vi "Demo_DatabaseTest_NIbase.vi"() -> ()   [LabVIEW 2016]
uses:
  <vilib>/addons/database/Connection.llb/DB Tools Open Connec (String).vi
  <vilib>/addons/database/Connection.llb/DB Tools Open Connec (Path).vi
  <vilib>/addons/database/Connection.llb/Conn Execute.vi
  <vilib>/addons/database/NI_Database_API.lvlib
panel:
  out "error out":errorcluster
  in  "msgid":dbl
  in  "content":string
  in  "dataLabel":string
  in  "TestId":string
  in  "错误输入 16":errorcluster caption="错误输入"
  in  "Connection Method":u16(ring) items=["ODBC System DSN", "UDL File", "Prompt"]
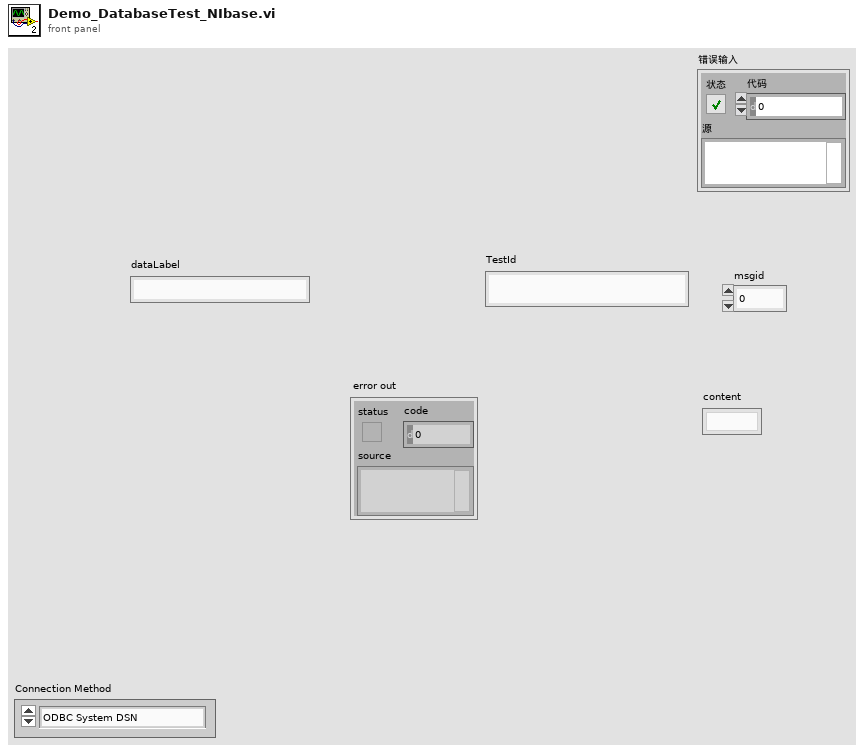
[diagram p1: front panel]
types:
  T1 = typedef "NI_Database_API.lvlib/Conn ObjectReference.ctl" = refnum<k1>
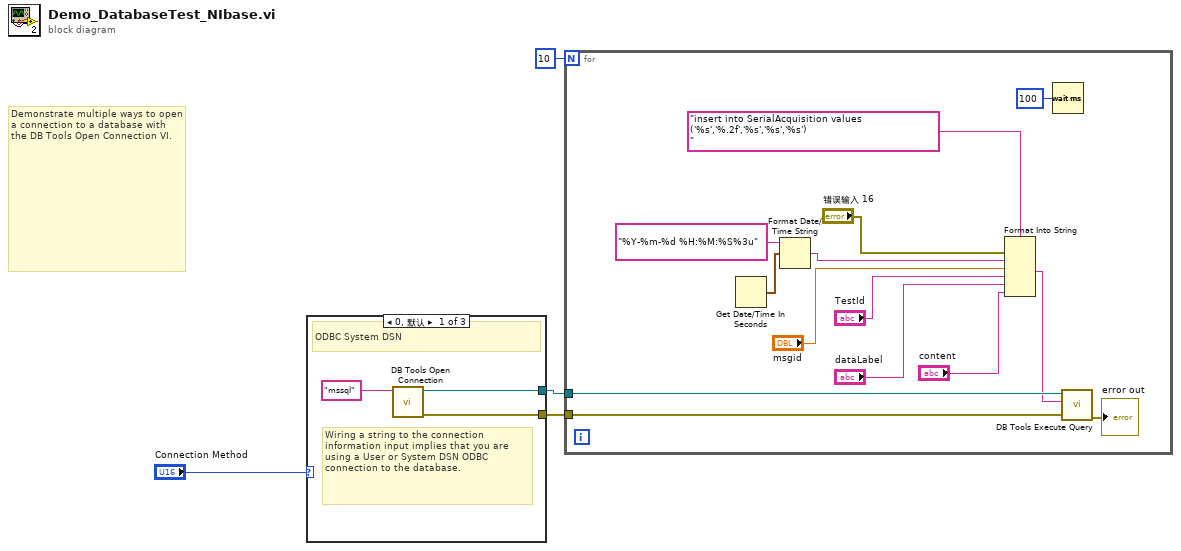
[diagram p0: block diagram]
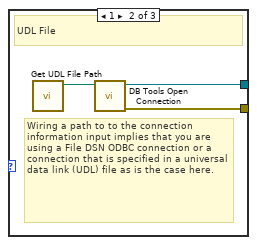
[diagram p2: hidden frame]
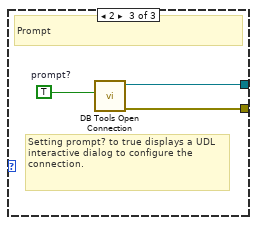
[diagram p3: hidden frame]
diagram:
  # "Demonstrate multiple ways to open a connection to a database with the DB Tools Open Connection VI."
  n1 = case shown="0, 默认" "Connection Method" {
    tunnel: [w6 w9 w13] -> w3
    tunnel: [w5 w10 w12] -> w2
    frame 0, Default {
      # "Wiring a string to the connection information input implies that you are using a User or System DSN ODBC connection to the database."
      # "ODBC System DSN"
      n2 = call-poly <vilib>:"DB Tools Open Connection.vi"("connection information"="mssql") -> ("error out"=w5:errorcluster, "connection reference"=w6:T1)  [unwired: 7 in]
    }
    frame 1 {
      # "Wiring a path to to the connection information input implies that you are using a File DSN ODBC connection or a connection that is specified in a universal data link (UDL) file as is the case here."
      # "UDL File"
      n3 = call "Get UDL File Path.vi"() -> ("UDL file path"=w8:path)  [unwired: 11 in]
      n4 = call-poly <vilib>:"DB Tools Open Connection.vi"("connection information"=w8) -> ("error out"=w10:errorcluster, "connection reference"=w9:T1)  [unwired: 7 in]
    }
    frame 2 {
      w11 = TRUE  # prompt?
      # "Setting prompt? to true displays a UDL interactive dialog to configure the connection."
      # "Prompt"
      n5 = call-poly <vilib>:"DB Tools Open Connection.vi"("prompt? (F)"=w11) -> ("error out"=w12:errorcluster, "connection reference"=w13:T1)  [unwired: 7 in]
    }
  }
  n6 = for {
    N: 10 -> [_]
    tunnel: w3 -> [w27]
    tunnel: w2 -> [w17]
    n7 = Get Date/Time In Seconds() -> (seconds since 1Jan1904=w24:timestamp)
    n8 = Format Date/Time String ("格式化日期/时间字符串")(time format string (%c)="%Y-%m-%d %H:%M:%S%3u" ("时间格式字符串(%c)"), seconds (now)=w24) -> (date/time string=w22:string)  [unwired: 1 in]
    n9 = Format Into String(format string="insert into SerialAcquisition values ('%s','%.2f','%s','%s','%s')                                                      " ("格式字符串"), error in="错误输入 16", w22, "msgid", "TestId", "dataLabel", "content") -> (resulting string=w16:string)  [unwired: 1 in, 1 out]
    n10 = Wait (ms)(milliseconds to wait=u32 100 ("等待时间（毫秒）")) -> ()  [unwired: 1 out]
    n11 = call-poly <vilib>:"DB Tools Execute Query.vi"("error in (no error)"=w17, "SQL query"=w16, "connection reference"=w27) -> ("error out"=→"error out":errorcluster)  [unwired: 5 in, 1 out]
  }
